vi "Tosca-DI Thread.vi"(0 "IPC":T1, 5 "Action":enum16{"Stop", "Preview", "Run"}(ring), 7 "Input Events":T3[](array[typedef])=[{"Name"="", "Criteria"=[{"DigInput"=1, "State"=enum."High", "Time (ms)"=500, "Name"=""}], "Operators"=[], "Accumulator"={"active"=FALSE, "N"=0, "T"=0.0, "Imax"=0.0, "latency"=0.0}}]) -> (15 "error out":errorcluster)   [LabVIEW 2020]
uses:
  Tosca-Input Event.ctl
  Tosca-Input Criterion.ctl
  epl-vi-lib/Utility VIs/Type Defs/Logic State.ctl
  Typedefs/Tosca-Accumulator.ctl
  IPC VIs/Tosca-IPC.ctl
  Classes/Parameters/Parameters.lvclass
  Tosca-DI Queue Data.ctl
  Typedefs/Tosca-State AODO.ctl
  Typedefs/Tosca-AO Runtime.ctl
  Typedefs/Tosca-DO Runtime.ctl
  epl-vi-lib/Signal Synthesis VIs/4th Generation/Classes/SignalManager/SignalManager.lvclass
  Typedefs/Tosca-Synapse Start Data.ctl
  IPC VIs/Tosca-Message.ctl
  IPC VIs/Tosca-Message Action.ctl
  Typedefs/Tosca-Thread Type.ctl
  Imaging VIs/Tosca-2P-Notifier Data.ctl
  Typedefs/Tosca-MATLAB Queue Data.ctl
  Visual Stim VIs/Tosca-Grating.ctl
  Visual Stim VIs/Tosca-Grating Type.ctl
  Typedefs/Tosca-File IO Notification.ctl
  Tosca-DI Write Data.ctl
  Tosca-DI Acq Data.ctl
panel:
  out "Overload":bool caption="overload"
  out "DI Indicators":T2
  out "Event Indicators":T2
  out "dt":i64=3 format="dt = %.0f ms"
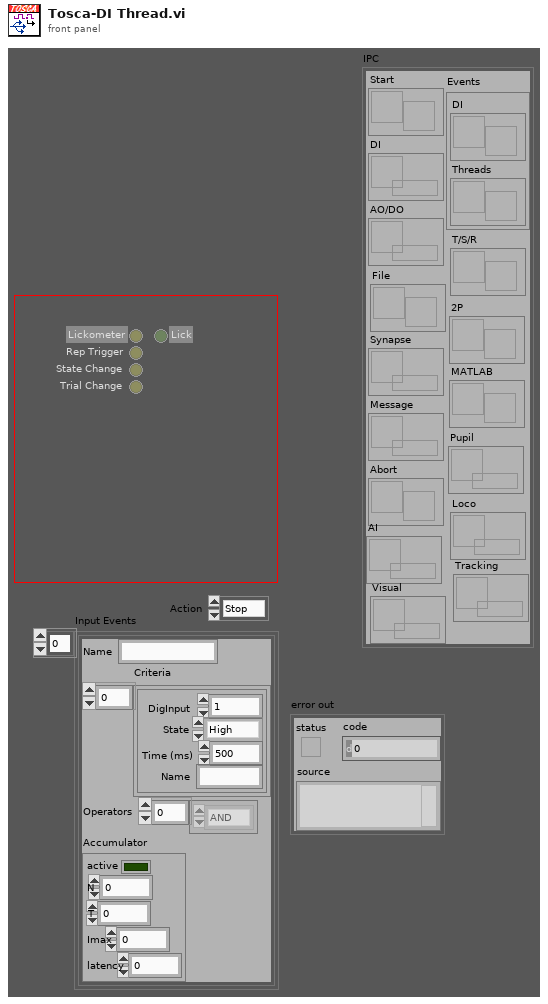
[diagram p1: front panel]
types:
  T1 = typedef "Tosca-IPC.ctl" = cluster{"Start":refnum<notifier>, "DI":refnum<queue>, "AO/DO":refnum<queue>, "Synapse":refnum<queue>, "Message":refnum<queue>, "Abort":refnum<notifier>, "Events":cluster{"DI":refnum<user-event>, "Threads ":refnum<user-event>}, "T/S/R":refnum<notifier>, "2P":refnum<notifier>, "MATLAB":refnum<notifier>, "Pupil":refnum<queue>, "Loco":refnum<queue>, "AI":refnum<queue>, "Tracking":refnum<queue>, "Visual":refnum<queue>, "File":refnum<notifier>}
  T2 = cluster{"Input 1":bool, "Input 2":bool, "Input 3":bool, "Input 4":bool, "Input 5":bool, "Input 6":bool, "Input 7":bool, "Input 8":bool}
  T3 = typedef "Tosca-Input Event.ctl" = cluster{"Name":string, "Criteria":T4[], "Operators":enum16{"AND", "OR"}[], "Accumulator":T6}
  T4 = typedef "Tosca-Input Criterion.ctl" = cluster{"DigInput":i32, "State":T5, "Time (ms)":i32, "Name":string}
  T5 = typedef "Logic State.ctl" = enum16{"Low", "High", "Rising", "Falling"}
  T6 = typedef "Tosca-Accumulator.ctl" = cluster{"active":bool, "N":i32, "T":dbl, "Imax":dbl, "latency":dbl}
  T7 = typedef "Tosca-Digital Input.ctl" = cluster{"Name":string, "State":bool, "Time (ms)":dbl, "Line":i32, "Rise":bool, "Fall":bool}
  T8 = typedef "Tosca-DI Write Data.ctl" = cluster{"loop time":dbl, "digital":bool[], "events":bool[], "last":bool, "time":dbl}
  T9 = typedef "Tosca-DI Acq Data.ctl" = cluster{"dt":i64, "loop":dbl, "digital":bool[], "events":bool[], "time":dbl, "overtime":bool}
  T10 = cluster{"digital[0]":bool, "digital[1]":bool, "digital[2]":bool, "digital[3]":bool, "digital[4]":bool, "digital[5]":bool, "digital[6]":bool, "digital[7]":bool}
  T11 = cluster{"events[0]":bool, "events[1]":bool, "events[2]":bool, "events[3]":bool, "events[4]":bool, "events[5]":bool, "events[6]":bool, "events[7]":bool}
  T12 = cluster{"loop":dbl, "digital":bool[], "events":bool[], bool, "time":dbl}
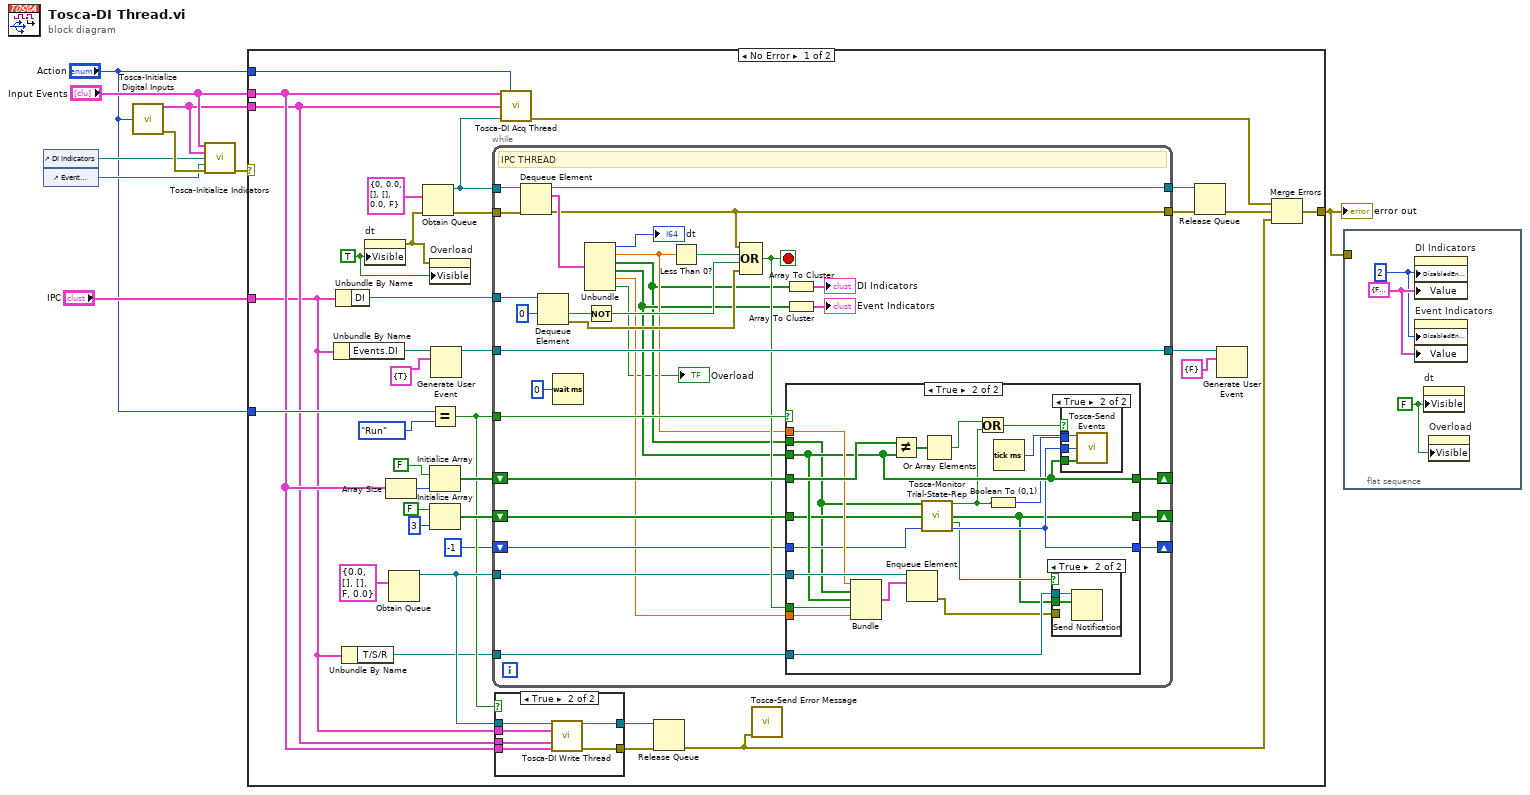
[diagram p0: block diagram]
diagram:
  n1 = control-ref of="DI Indicators"() -> (w4:refnum<vi>)
  n2 = control-ref of="Event Indicators"() -> (w3:refnum<vi>)
  n3 = call "Tosca-Initialize Digital Inputs.vi"("Action"="Action") -> ("Digital Inputs out"=w5:T7[], "error out"=w9:errorcluster)  [unwired: 13 in]
  n4 = call "Tosca-Initialize Indicators.vi"("Input Events"="Input Events", "Digital Inputs"=w5, "DI Indicators"=w4, "Event Indicators"=w3, "error in (no error)"=w9) -> ("error out"=w7:errorcluster)  [unwired: 10 in]
  n5 = case shown="No Error" w7 {
    selector: w7 -> [_ w113]
    tunnel: [w38 w113] -> w1
    tunnel: "IPC" -> [w19 _]
    tunnel: "Action" -> [w34 _]
    tunnel: "Input Events" -> [w25 _]
    tunnel: w5 -> [w24 _]
    tunnel: "Action" -> [w17 _]
    frame No Error {
      w12 = TRUE ("Visible")
      n6 = Unbundle By Name(w19) -> ("Events.DI"=w36:refnum<user-event>)
      n7 = Unbundle By Name(w19) -> ("DI"=w40:refnum<queue>)
      n8 = Unbundle By Name(w19) -> ("T/S/R"=w18:refnum<notifier>)
      n9 = property on="dt" class="DigNum (strict)"("Visible"=w12) -> (error out=w11:errorcluster)  [unwired: 2 in, 1 out]
      n10 = Array Size(array=w25) -> (size(s)=w43:i32)
      n11 = Obtain Queue(element data type=T8 {"loop time"=0.0, "digital"=[], "events"=[], "last"=FALSE, "time"=0.0} ("output cluster")) -> (queue out=w27:refnum<queue>)  [unwired: 4 in, 2 out]
      n12 = Obtain Queue(element data type=T9 {"dt"=0, "loop"=0.0, "digital"=[], "events"=[], "time"=0.0, "overtime"=FALSE} ("output cluster"), error in (no error)=w11) -> (queue out=w23:refnum<queue>, error out=w44:errorcluster)  [unwired: 3 in, 1 out]
      n13 = property on="Overload" class="Bool (strict)"(error in=w11, "Visible"=w12) -> ()  [unwired: 1 in, 2 out]
      n14 = Equal?(x=w34, y=enum16{"Stop", "Preview", "Run"}."Run") -> (x = y?=w26:bool)
      n15 = Initialize Array(FALSE, w43) -> (w41:bool[])
      n16 = Initialize Array(FALSE, 3 ("dimension size")) -> (w30:bool[])
      n17 = Generate User Event(user event=w36, event data cluster=cluster{"Running":bool} {"Running"=TRUE} ("event data")) -> (user event out=w35:refnum<user-event>)  [unwired: 2 in, 1 out]
      n18 = while {
        tunnel: w23 -> [w76]
        tunnel: [w49] -> w16
        tunnel: w44 -> [w73]
        tunnel: [w68] -> w15
        shift-right: [w62] -> _
        shift-left: w41 -> [w63]
        tunnel: w40 -> [w71]
        tunnel: w35 -> [w65]
        tunnel: [w65] -> w14
        tunnel: w26 -> [w64]
        shift-right: [w60] -> _
        shift-left: w30 -> [w61]
        tunnel: w27 -> [w58]
        shift-right: [w52] -> _
        shift-left: -1 -> [w53]
        tunnel: w18 -> [w51]
        stop <- w59 stop-if-true
        # "IPC THREAD"
        n19 = Dequeue Element(queue=w76, error in (no error)=w73) -> (queue out=w49:refnum<queue>, element=w75:T9, error out=w68:errorcluster)  [unwired: 1 in, 1 out]
        n20 = Dequeue Element(queue=w71, timeout in ms (-1)=0) -> (timed out?=w69:bool, error out=w66:errorcluster)  [unwired: 1 in, 2 out]
        n21 = Wait (ms)(milliseconds to wait=u32 0) -> ()  [unwired: 1 out]
        n22 = Unbundle(w75) -> ("dt"=→"dt":i64, "loop"=w57:dbl, "digital"=w55:bool[], "events"=w56:bool[], "time"=w48:dbl, "overtime"=→"Overload":bool)
        n23 = Not(x=w69) -> (.not. x?=w67:bool)
        n24 = Less Than 0?(x=w57) -> (x < 0?=w72:bool)
        n25 = Compound Arithmetic op=OR(w68, w72, w67, w66) -> (w59:bool)
        n26 = Array To Cluster(array=w55) -> (cluster=→"DI Indicators":T10)
        n27 = Array To Cluster(array=w56) -> (cluster=→"Event Indicators":T11)
        n28 = case shown="True" w64 {
          tunnel: w63 -> [w79 w98]
          tunnel: [w79 w93] -> w62
          tunnel: w61 -> [w78 w91]
          tunnel: [w78 w84] -> w60
          tunnel: w57 -> [_ w97]
          tunnel: w59 -> [_ w96]
          tunnel: w55 -> [_ w89]
          tunnel: w56 -> [_ w93]
          tunnel: w58 -> [_ w100]
          tunnel: w53 -> [w77 w90]
          tunnel: [w77 w88] -> w52
          tunnel: w51 -> [_ w85]
          tunnel: w48 -> [_ w82]
          frame False {
          }
          frame True {
            n29 = Bundle("loop"=w97, "digital"=w89, "events"=w93, w96, "time"=w82) -> (w95:T12)  [unwired: 1 in]
            n30 = Not Equal?(x=w98, y=w93) -> (x != y?=w99:bool[])
            n31 = Enqueue Element(queue=w100, element=w95) -> (error out=w83:errorcluster)  [unwired: 2 in, 2 out]
            n32 = call "Tosca-Monitor Trial-State-Rep.vi"("DI"=w89, "Trial/State/Rep In"=w91, "State In"=w90) -> ("State change?"=w81:bool, "Trial/State/Rep Out"=w84:bool[], "Any change"=w86:bool, "State Out"=w88:i32)  [unwired: 9 in]
            n33 = Or Array Elements(Boolean array=w99) -> (logical OR=w92:bool)
            n34 = Or(x=w92, y=w81) -> (x .or. y?=w87:bool)
            n35 = Boolean To (0,1)(Boolean=w81) -> (0, 1=w80:i16)
            n36 = Tick Count (ms)() -> (millisecond timer value=w94:u32)
            n37 = case shown="True" w86 {
              tunnel: w85 -> [_ w102]
              tunnel: w84 -> [_ w101]
              tunnel: w83 -> [_ _]
              frame False {
              }
              frame True {
                n38 = Send Notification(notification=w101, notifier=w102) -> ()  [unwired: 1 in, 2 out]
              }
            }
            n39 = case shown="True" w87 {
              tunnel: w94 -> [_ w105]
              tunnel: w88 -> [_ w104]
              tunnel: w93 -> [_ w103]
              tunnel: w80 -> [_ _]
              frame False {
              }
              frame True {
                n40 = call "Tosca-Send Events.vi"("Time"=w105, "State"=w104, "Events"=w103) -> ()  [unwired: 13 in]
              }
            }
          }
        }
      }
      n41 = case shown="True" w26 {
        tunnel: [_ w112] -> w21
        tunnel: w24 -> [_ w110]
        tunnel: w25 -> [_ w109]
        tunnel: w27 -> [w106 w111]
        tunnel: w19 -> [_ w108]
        tunnel: [w106 w107] -> w22
        frame False {
        }
        frame True {
          n42 = call "Tosca-DI Write Thread.vi"("Write Data"=w111, "IPC"=w108, "Digital Inputs"=w110, "Input Events"=w109) -> ("Write Data thru"=w107:refnum<queue>, "error out"=w112:errorcluster)  [unwired: 10 in]
        }
      }
      n43 = call "Tosca-DI Acq Thread.vi"("Input Events"=w25, "Action"=w17, "Digital Inputs in"=w24, "Acq Data"=w23) -> ("error out"=w28:errorcluster)  [unwired: 11 in]
      n44 = Release Queue(queue=w22, error in (no error)=w21) -> (error out=w10:errorcluster)  [unwired: 1 in, 2 out]
      n45 = call "Tosca-Send Error Message.vi"("error in (no error)"=w10) -> ()  [unwired: 15 in]
      n46 = Release Queue(queue=w16, error in (no error)=w15) -> (error out=w39:errorcluster)  [unwired: 1 in, 2 out]
      n47 = Generate User Event(user event=w14, event data cluster=cluster{"Running":bool} {"Running"=FALSE} ("event data")) -> ()  [unwired: 2 in, 2 out]
      n48 = Merge Errors(w28, w39, w10) -> (w38:errorcluster)
    }
    frame Error {
    }
  }
  "error out" <- w1
  n49 = flat-sequence {
    tunnel: w1 -> [_]
    frame #0 {
      w116 = T2 {"Input 1"=FALSE, "Input 2"=FALSE, "Input 3"=FALSE, "Input 4"=FALSE, "Input 5"=FALSE, "Input 6"=FALSE, "Input 7"=FALSE, "Input 8"=FALSE} ("DI Indicators")
      w115 = 2
      w114 = FALSE
      n50 = property on="DI Indicators" class="Clust (strict)"("DisabledEnum"=w115, "Value"=w116) -> ()  [unwired: 2 in, 2 out]
      n51 = property on="Event Indicators" class="Clust (strict)"("DisabledEnum"=w115, "Value"=w116) -> ()  [unwired: 2 in, 2 out]
      n52 = property on="dt" class="DigNum (strict)"("Visible"=w114) -> ()  [unwired: 2 in, 2 out]
      n53 = property on="Overload" class="Bool (strict)"("Visible"=w114) -> ()  [unwired: 2 in, 2 out]
    }
  }
